vi "set group.vi"(0 "VISA in":refnum<visa-resource-name>, 1 "Location Cluster in":T1, 4 "Group":string, 5 "error in (no error)":errorcluster) -> (14 "VISA out":refnum<visa-resource-name>, 15 "Location Cluster out":T1, 19 "error out":errorcluster)   [LabVIEW 2018]
uses:
  location cluster.ctl
  CAEN globals.vi
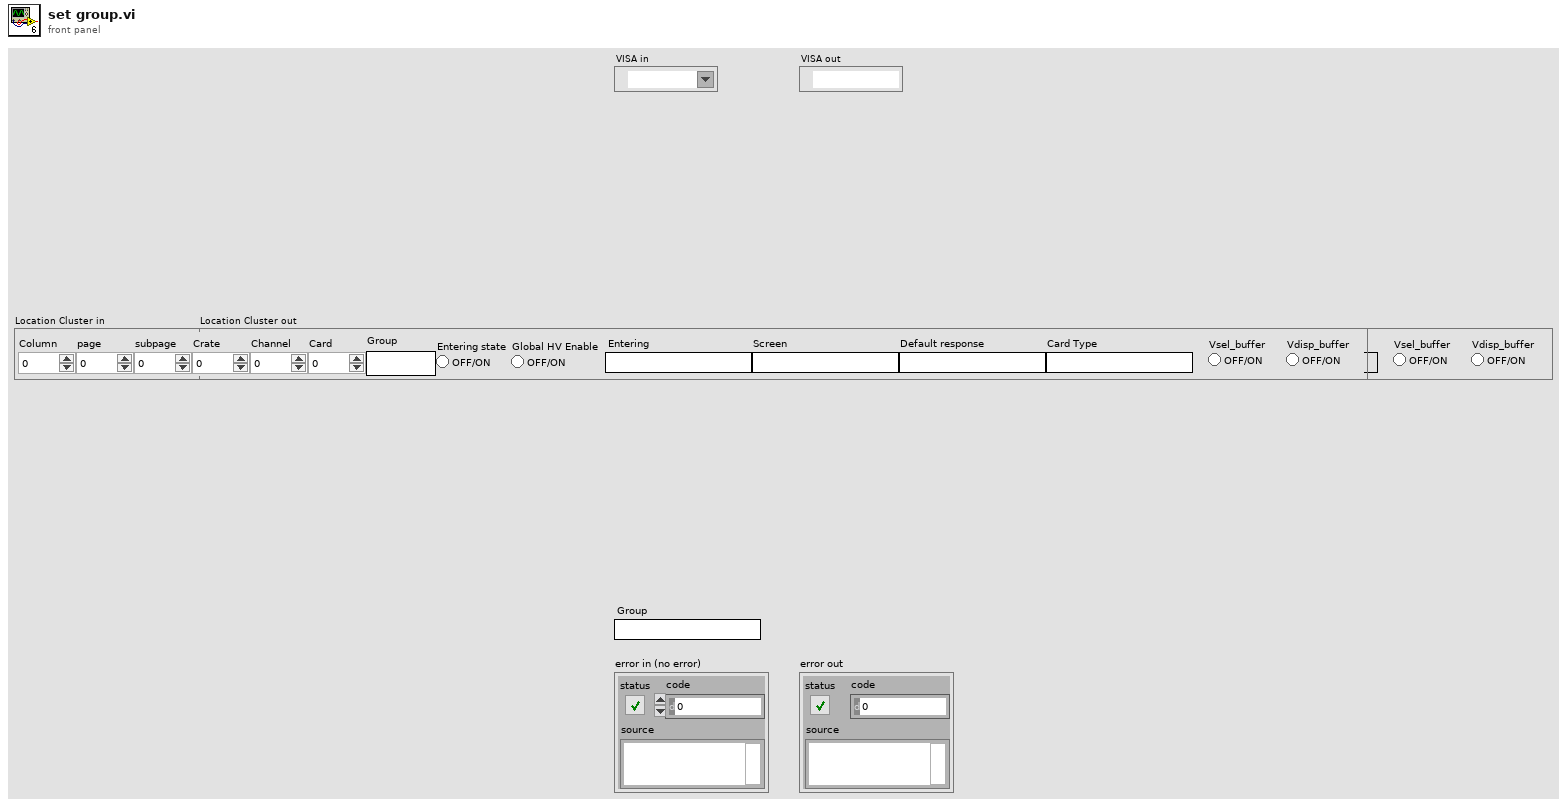
[diagram p1: front panel]
types:
  T1 = typedef "location cluster.ctl" = cluster{"Column":i32, "Card Type":string, "Channel":i32, "Card":i32, "Default response":string, "Entering":string, "Entering state":bool, "subpage":i32, "page":i32, "Crate":i32, "Screen":string, "Group":string, "Global HV Enable":bool, "Vsel_buffer":bool, "Vdisp_buffer":bool}
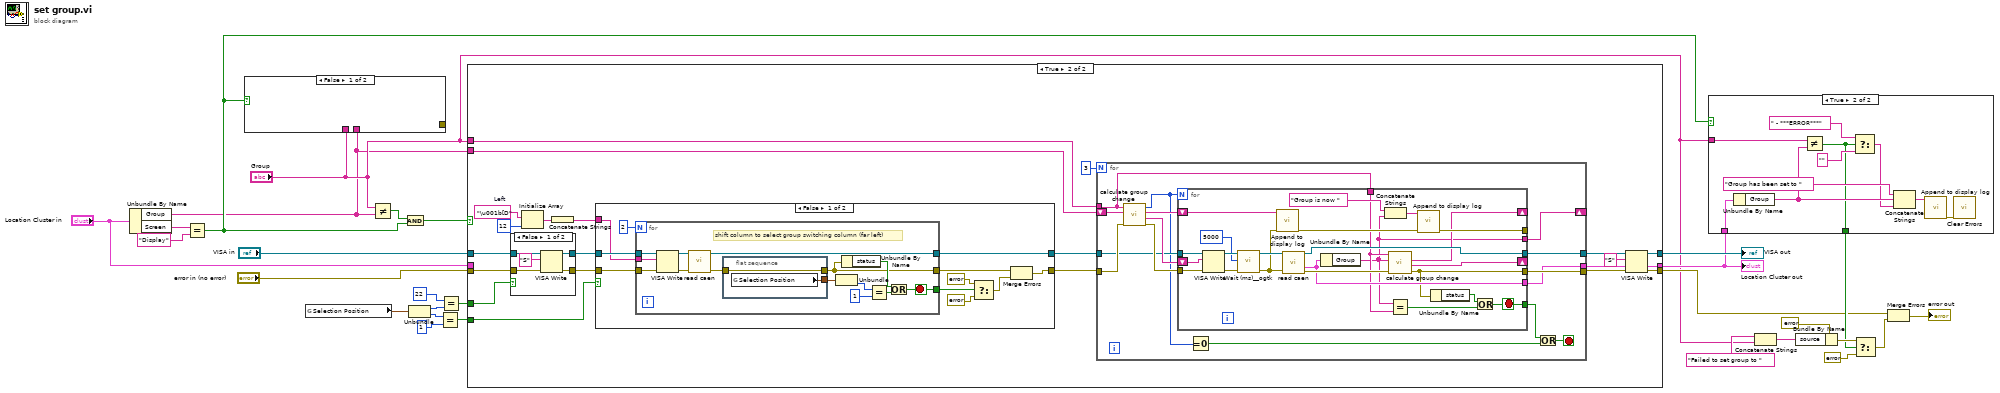
[diagram p0: block diagram]
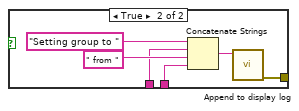
[diagram p3: hidden frame]
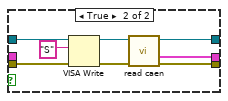
[diagram p5: hidden frame]
diagram:
  n1 = Unbundle By Name("Location Cluster in") -> ("Group"=w9:string, "Screen"=w25:string)
  n2 = Equal?(x=w25, y="Display" ("x")) -> (x = y?=w11:bool)
  n3 = case shown="False" w11 {
    tunnel: [_ w31] -> _
    tunnel: w9 -> [_ w30]
    tunnel: "Group" -> [_ w29]
    frame False {
    }
    frame True {
      n4 = Concatenate Strings("Setting group to " ("string"), w29, " from " ("string"), w30) -> (w33:string)
      n5 = call "Append to display log.vi"("string"=w33) -> ("error out"=w31:errorcluster)  [unwired: 10 in]
    }
  }
  n6 = global read "CAEN globals.vi" "Selection Position"() -> (w3:cluster{i32, i32})
  n7 = Not Equal?(x="Group", y=w9) -> (x != y?=w23:bool)
  n8 = And(x=w23, y=w11) -> (x .and. y?=w22:bool)
  n9 = Unbundle(w3) -> (w4:i32, w5:i32)
  n10 = Equal?(x=w5, y=1 ("x")) -> (x = y?=w1:bool)
  n11 = Equal?(x=22, y=w4) -> (x = y?=w2:bool)
  n12 = case shown="True" w22 {
    tunnel: "error in (no error)" -> [w39 w72]
    tunnel: "Location Cluster in" -> [w37 _]
    tunnel: "VISA in" -> [w41 w73]
    tunnel: "Group" -> [_ w65]
    tunnel: [w40 w58] -> w28
    tunnel: [w36 w64] -> w14
    tunnel: [w38 w59] -> w13
    tunnel: w9 -> [_ w53]
    tunnel: w2 -> [w35 w57]
    tunnel: w1 -> [_ w56]
    frame False {
      n13 = case shown="False" w35 {
        tunnel: w41 -> [w44 w52]
        tunnel: w39 -> [w43 w51]
        tunnel: [w43 w47] -> w38
        tunnel: [w44 w46] -> w40
        tunnel: w37 -> [w42 _]
        tunnel: [w42 w45] -> w36
        frame False {
        }
        frame True {
          n14 = VISA Write(VISA resource name=w52, write buffer="S", error in (no error)=w51) -> (VISA resource name out=w48:refnum<visa-resource-name>, error out=w49:errorcluster)  [unwired: 1 out]
          n15 = call "read caen.vi"("VISA in"=w48, "error in"=w49) -> ("VISA out"=w46:refnum<visa-resource-name>, "Location Cluster"=w45:T1, "error out"=w47:errorcluster)  [unwired: 8 in, 3 out]
        }
      }
    }
    frame True {
      w67 = "\u001b[D"  # Left
      n16 = case shown="False" w57 {
        tunnel: w73 -> [w145 w147]
        tunnel: w72 -> [w144 w146]
        tunnel: [w142 w146] -> w70
        tunnel: [w141 w147] -> w71
        frame False {
          n17 = VISA Write(VISA resource name=w145, write buffer="S", error in (no error)=w144) -> (VISA resource name out=w141:refnum<visa-resource-name>, error out=w142:errorcluster)  [unwired: 1 out]
        }
        frame True {
        }
      }
      n18 = Initialize Array(w67, 12 ("dimension size")) -> (w69:string[])
      n19 = Concatenate Strings(w69) -> (w66:string)
      n20 = case shown="False" w56 {
        tunnel: w71 -> [w122 w140]
        tunnel: w70 -> [w121 w139]
        tunnel: [w113 w139] -> w54
        tunnel: [w112 w140] -> w55
        tunnel: w66 -> [w120 _]
        frame False {
          n21 = for {
            N: 2 -> [_]
            tunnel: w122 -> [w136]
            tunnel: w121 -> [w135]
            tunnel: w120 -> [w134]
            tunnel: [w127] -> w117
            tunnel: [w123] -> w114
            tunnel: [w126] -> w112
            stop <- w127 stop-if-true
            # "shift column to select group switching column (far left)"
            n22 = VISA Write(VISA resource name=w136, write buffer=w134, error in (no error)=w135) -> (VISA resource name out=w133:refnum<visa-resource-name>, error out=w132:errorcluster)  [unwired: 1 out]
            n23 = call "read caen.vi"("VISA in"=w133, "error in"=w132) -> ("VISA out"=w126:refnum<visa-resource-name>, "error out"=w124:errorcluster)  [unwired: 8 in, 4 out]
            n24 = flat-sequence {
              tunnel: [w138] -> w125
              tunnel: [w137] -> w123
              tunnel: w124 -> [w137]
              frame #0 {
                n25 = global read "CAEN globals.vi" "Selection Position"() -> (w138:cluster{i32, i32})
              }
            }
            n26 = Unbundle(w125) -> (w130:i32)  [unwired: 1 out]
            n27 = Unbundle By Name(w123) -> ("status"=w128:bool)
            n28 = Equal?(x=w130, y=1 ("x")) -> (x = y?=w129:bool)
            n29 = Or(x=w128, y=w129) -> (x .or. y?=w127:bool)
          }
          n30 = Select(t=errorcluster {"status"=FALSE, "code"=0, "source"=""}, s=w117, f=errorcluster {"status"=TRUE, "code"=0, "source"="Failed to select group editing column"} ("error out")) -> (s? t:f=w115:errorcluster)
          n31 = Merge Errors(w114, w115) -> (w113:errorcluster)
        }
        frame True {
        }
      }
      n32 = for {
        N: 3 -> [_]
        tunnel: w65 -> [w79]
        tunnel: [w80] -> w64
        tunnel: w55 -> [w84]
        tunnel: [w82] -> w61
        tunnel: w54 -> [w88]
        tunnel: [w81] -> w60
        shift-right: [w78] -> _
        shift-left: w53 -> [w83]
        stop <- w74 stop-if-true
        n33 = call "calculate group change.vi"("error in"=w88, "Current group"=w83, "Set group"=w79) -> ("error out"=w85:errorcluster, "keystroke"=w86:string, "Action"=w87:string, "num changes"=w77:i32)  [unwired: 5 in]
        n34 = for {
          N: w77 -> [_]
          shift-right: [w99] -> _
          shift-left: w87 -> [w108]
          shift-right: [w98] -> _
          shift-left: w86 -> [w109]
          tunnel: w85 -> [w110]
          tunnel: w84 -> [w111]
          tunnel: w79 -> [w96]
          tunnel: [w103] -> w82
          tunnel: [w97] -> w81
          tunnel: [w102] -> w80
          tunnel: [w100] -> _
          tunnel: [w93] -> w75
          tunnel: [w92] -> w78
          stop <- w93 stop-if-true
          n35 = VISA Write(VISA resource name=w111, write buffer=w109, error in (no error)=w110) -> (VISA resource name out=w107:refnum<visa-resource-name>, error out=w91:errorcluster)  [unwired: 1 out]
          n36 = call <userlib>:"Wait (ms)__ogtk.vi"("error in (no error)"=w91, "milliseconds to wait"=u32 5000) -> ("error out"=w90:errorcluster)  [unwired: 8 in, 1 out]
          n37 = call "Append to display log.vi"("error in"=w90, "string"=w108) -> ("error out"=w101:errorcluster)  [unwired: 9 in]
          n38 = call "read caen.vi"("VISA in"=w107, "error in"=w90) -> ("VISA out"=w103:refnum<visa-resource-name>, "Location Cluster"=w102:T1, "error out"=w106:errorcluster)  [unwired: 8 in, 3 out]
          n39 = Unbundle By Name(w102) -> ("Group"=w92:string)
          n40 = Concatenate Strings("Group is now " ("string"), w92) -> (w105:string)
          n41 = call "calculate group change.vi"("error in"=w106, "Current group"=w92, "Set group"=w96) -> ("error out"=w97:errorcluster, "keystroke"=w98:string, "Action"=w99:string)  [unwired: 5 in, 1 out]
          n42 = Equal?(x=w92, y=w96) -> (x = y?=w94:bool)
          n43 = call "Append to display log.vi"("error in"=w101, "string"=w105) -> ("error out"=w100:errorcluster)  [unwired: 9 in]
          n44 = Unbundle By Name(w97) -> ("status"=w95:bool)
          n45 = Or(x=w95, y=w94) -> (x .or. y?=w93:bool)
        }
        n46 = Equal To 0?(x=w77) -> (x = 0?=w76:bool)
        n47 = Or(x=w75, y=w76) -> (x .or. y?=w74:bool)
      }
      n48 = VISA Write(VISA resource name=w61, write buffer="S", error in (no error)=w60) -> (VISA resource name out=w58:refnum<visa-resource-name>, error out=w59:errorcluster)  [unwired: 1 out]
    }
  }
  "Location Cluster out" <- w14
  "VISA out" <- w28
  n49 = case shown="True" w11 {
    tunnel: [_ w150] -> w17
    tunnel: w14 -> [_ w149]
    tunnel: "Group" -> [_ w148]
    frame False {
    }
    frame True {
      n50 = Unbundle By Name(w149) -> ("Group"=w152:string)
      n51 = Not Equal?(x=w148, y=w152) -> (x != y?=w150:bool)
      n52 = Select(t=" - ***ERROR***" ("string"), s=w150, f="" ("string")) -> (s? t:f=w151:string)
      n53 = Concatenate Strings("Group has been set to " ("string"), w152, w151) -> (w157:string)
      n54 = call "Append to display log.vi"("string"=w157) -> ("error out"=w155:errorcluster)  [unwired: 10 in]
      n55 = call <vilib>:"Clear Errors.vi"("error in (no error)"=w155) -> ()  [unwired: 5 in, 2 out]
    }
  }
  n56 = Concatenate Strings("Failed to set group to " ("string"), "Group") -> (w16:string)
  n57 = Bundle By Name(cluster=errorcluster {"status"=TRUE, "code"=0, "source"=""} ("input cluster"), "source"=w16) -> (w18:errorcluster)
  n58 = Select(t=w18, s=w17, f=errorcluster {"status"=FALSE, "code"=0, "source"=""}) -> (s? t:f=w20:errorcluster)
  n59 = Merge Errors(w13, w20) -> (→"error out":errorcluster)
